vi "getVariaModuleType.vi"(8 "error in (no error)":errorcluster, 11 "VISA Refnum in":refnum<visa-resource-name>) -> (0 "error out":errorcluster, 2 "moduleType":i32 format="%x", 3 "VISA Refnum out":refnum<visa-resource-name>)   [LabVIEW 2014]
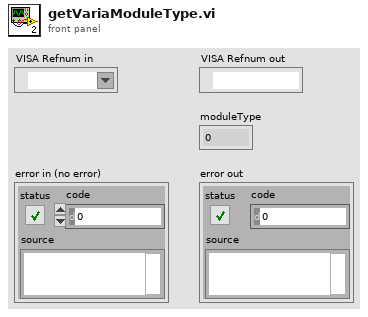
[diagram p1: front panel]
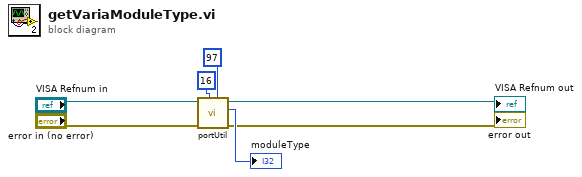
[diagram p0: block diagram]
diagram:
  n1 = call "portUtil.vi"("Register"=u8 97, "Destination"=u8 16, "error in (no error)"="error in (no error)", "VISA Refnum in"="VISA Refnum in") -> ("error out"=→"error out":errorcluster, "Long"=→"moduleType":i32, "VISA Refnum out"=→"VISA Refnum out":refnum<visa-resource-name>)  [unwired: 4 in, 1 out]
